vi "取消.vi"(8 "error in (no error)":errorcluster caption="错误输入（无错误）", 11 "命令：关闭冷却 输入":refnum<class "命令：关闭冷却.lvclass"> caption="DNL_LabVIEW Object in") -> (0 "error out":errorcluster caption="错误输出", 3 "命令：关闭冷却 输出":refnum<class "命令：关闭冷却.lvclass"> caption="DNL_LabVIEW Object out")   [LabVIEW 2011, in "命令：关闭冷却.lvclass"]
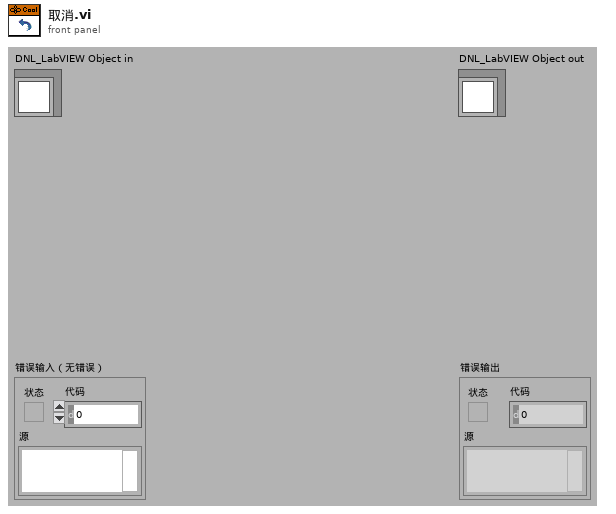
[diagram p1: front panel]
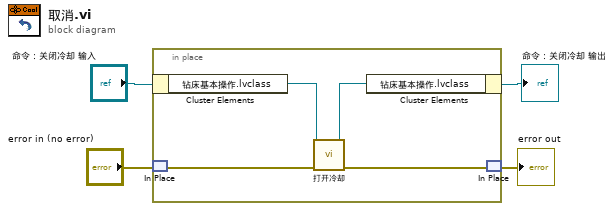
[diagram p0: block diagram]
diagram:
  n1 = in-place {
    n2 = in-place-cluster #1("命令：关闭冷却 输入") -> ("钻床基本操作.lvclass"=w8:refnum<class "钻床基本操作.lvclass">)
    n3 = in-place-match #2("error in (no error)") -> (w7:errorcluster)
    n4 = call "打开冷却.vi"("error in (no error)"=w7, "钻床基本操作 输入"=w8) -> ("error out"=w5:errorcluster, "钻床基本操作 输出"=w6:refnum<class "钻床基本操作.lvclass">)  [unwired: 8 in]
    n5 = in-place-cluster #1("钻床基本操作.lvclass"=w6) -> (→"命令：关闭冷却 输出":refnum<class "命令：关闭冷却.lvclass">)
    n6 = in-place-match #2(w5) -> (→"error out":errorcluster)
  }
